vi "Find Fiducials.vi"(7 "Console Log in":refnum<class "Console Log.lvclass">, 8 "error in":errorcluster, 11 "Potting Procedure in":refnum<class "Potting Procedure.lvclass">) -> (0 "error out":errorcluster, 3 "Potting Procedure out":refnum<class "Potting Procedure.lvclass">, 5 "Console Log out":refnum<class "Console Log.lvclass">)   [LabVIEW 2011, in "Potting Procedure.lvclass"]
uses:
  Potting Procedure.lvclass
  UI Classes/Console Log/Console Log.lvclass
  Shared Components/Utils/Type Definitions/Fiducial Image.ctl
  Shared Components/Utils/Type Definitions/Physical Image.ctl
  Shared Components/Vec3d Class/Vec3d Class.lvclass
  <vilib>/vision/Image Controls.llb/IMAQ Image.ctl
  Shared Components/Utils/Type Definitions/Fiducial with Source.ctl
  Type Definitions/Find Fiducials.ctl
  Potting Procedure.lvclass/Potting Procedure.ctl
  Shared Components/Gantry Class/Gantry Class.lvclass
  Shared Components/WorkTable Class/WorkTable Class.lvclass
  Shared Components/CameraTool Class/CameraTool Class.lvclass
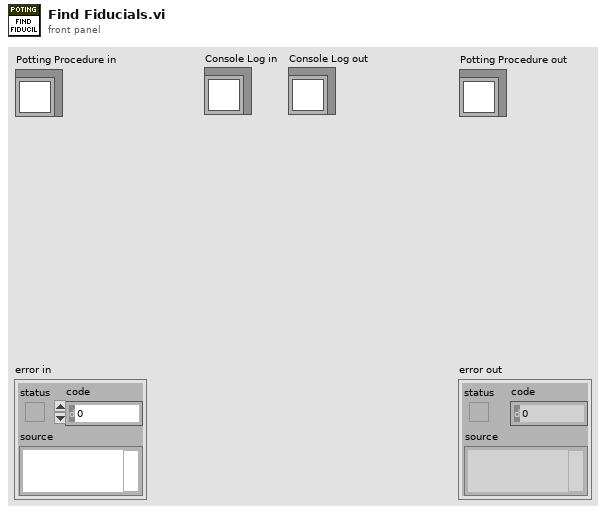
[diagram p1: front panel]
types:
  T1 = typedef "Fiducial Image.ctl" = cluster{"Fiducial Image":T2, "Selected Fiducial":T4}
  T2 = typedef "Physical Image.ctl" = cluster{"Image Position":refnum<class "Vec3d Class.lvclass">, "Image Reference":T3, "Field of View":cluster{"x(mm)":dbl, "y(mm)":dbl}}
  T3 = typedef "IMAQ Image.ctl" = refnum<image>
  T4 = typedef "Fiducial with Source.ctl" = cluster{"Fiducial Image Coordinate":refnum<class "Vec3d Class.lvclass">, "Fiducial Source":enum16{"Pattern Recognition", "User", "Error"}}
  T5 = cluster{"Fiducials-HDI":T1[], "Fiducials-BBM":T1[], "Chuck":i32, "Slot":i32}[]
  T6 = typedef "Find Fiducials.ctl" = cluster{"Has Been Run?":bool, "Module-Chuck Fiducials":cluster{"Fiducials-HDI":T1[], "Fiducials-BBM":T1[], "Chuck":i32, "Slot":i32}[]}
  T7 = enum16{"Empty", "Unglued", "Stamped", "PartOnTop", "Weighted", "Unpotted", "Potted"}
  T8 = cluster{"Fiducials-HDI":T1[], "Fiducials-BBM":T1[], "Chuck":i32, "Slot":i32}
  T9 = typedef "Worktable_Module Slot.ctl" = cluster{"Slot State":enum16{"Empty", "Unglued", "Stamped", "PartOnTop", "Weighted", "Unpotted", "Potted"}, "BBM Type":enum16{"None", "BBM", "GlassSlide"}, "HDI Type":enum16{"None", "HDI", "Polyimide"}, "Vacuum Channel":u8, "Location/Orientation BBM":T10, "Location/Orientation HDI":T10, "S/N":string}
  T10 = typedef "Position_Orientation.ctl" = cluster{"Center":refnum<class "Vec3d Class.lvclass">, "Orientation":refnum<class "Orient3d Class.lvclass">}
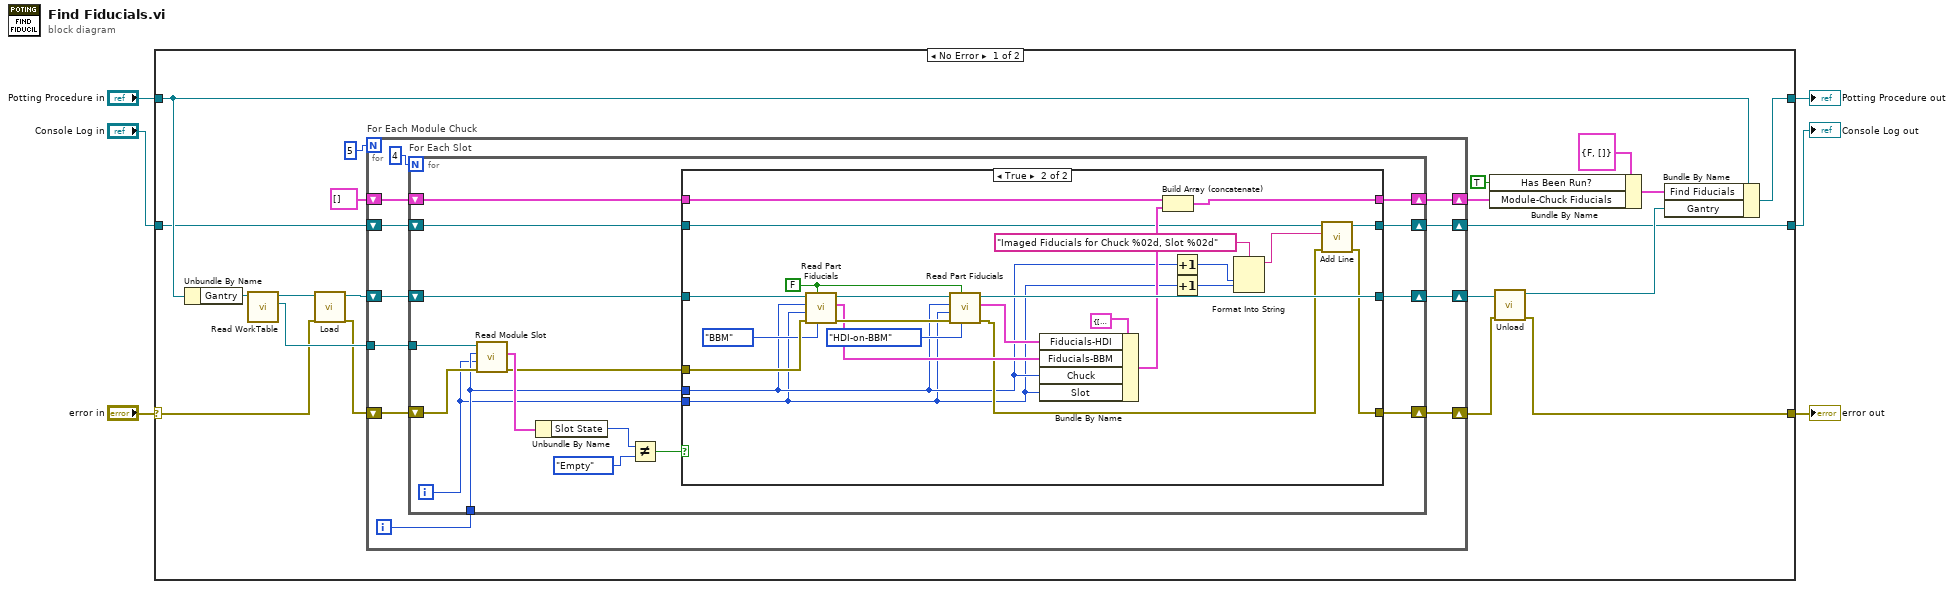
[diagram p0: block diagram]
diagram:
  n1 = case shown="No Error" "error in" {
    selector: "error in" -> [w18 w84]
    tunnel: [w14 w84] -> w5
    tunnel: [w13 w83] -> w3
    tunnel: "Potting Procedure in" -> [w16 w83]
    tunnel: "Console Log in" -> [w10 w82]
    tunnel: [w9 w82] -> w1
    frame No Error {
      n2 = Unbundle By Name(w16) -> ("Gantry"=w26:refnum<class "Gantry Class.lvclass">)
      n3 = call-dynamic "Read WorkTable.vi"("Gantry Class in"=w26) -> ("WorkTable Class.lvclass"=w24:refnum<class "WorkTable Class.lvclass">, "Gantry Class out"=w25:refnum<class "Gantry Class.lvclass">)  [unwired: 8 in, 1 out]
      n4 = call "Load.vi"("error in"=w18, "Gantry In"=w25) -> ("error out"=w22:errorcluster, "CameraTool out"=w21:refnum<class "CameraTool Class.lvclass">)  [unwired: 8 in]
      n5 = for "For Each Module Chuck" {
        N: 5 -> [_]
        tunnel: w24 -> [w37]
        shift-right: [w32] -> w17
        shift-left: w21 -> [w33]
        shift-right: [w31] -> w15
        shift-left: w22 -> [w35]
        shift-right: [w29] -> w7
        shift-left: T5 [] ("Module-Chuck Fiducials") -> [w30]
        shift-right: [w27] -> w9
        shift-left: w10 -> [w28]
        i -> [w34]
        n6 = for "For Each Slot" {
          N: 4 -> [_]
          tunnel: w37 -> [w53]
          tunnel: w34 -> [w46]
          shift-right: [w43] -> w32
          shift-left: w33 -> [w47]
          shift-right: [w42] -> w31
          shift-left: w35 -> [w52]
          shift-right: [w40] -> w29
          shift-left: w30 -> [w41]
          shift-right: [w38] -> w27
          shift-left: w28 -> [w39]
          i -> [w45]
          n7 = call-dynamic "Read Module Slot.vi"("error in"=w52, "slot"=w45, "chuck"=w46, "WorkTable in"=w53) -> ("error out"=w44:errorcluster, "Module Slot"=w51:T9)  [unwired: 5 in, 1 out]
          n8 = Unbundle By Name(w51) -> ("Slot State"=w49:T7)
          n9 = Not Equal?(x=w49, y=T7."Empty" ("BBM Slot State")) -> (x != y?=w48:bool)
          n10 = case shown="True" w48 {
            tunnel: w47 -> [w57 w81]
            tunnel: w46 -> [_ w60]
            tunnel: w45 -> [_ w59]
            tunnel: w44 -> [w56 w80]
            tunnel: [w57 w72] -> w43
            tunnel: [w56 w65] -> w42
            tunnel: w41 -> [w55 w71]
            tunnel: [w55 w69] -> w40
            tunnel: w39 -> [w54 w68]
            tunnel: [w54 w67] -> w38
            frame False {
            }
            frame True {
              w77 = FALSE ("Dispose Images?")
              n11 = call-dynamic "Read Part Fiducials.vi"("Part Type"=enum16{"HDI", "BBM", "HDI-on-BBM"}."BBM", "Dispose Images?"=w77, "error in"=w80, "Slot"=w59, "Chuck"=w60, "CameraTool in"=w81) -> ("error out"=w76:errorcluster, "Fiducials"=w73:T1[], "CameraTool out"=w78:refnum<class "CameraTool Class.lvclass">)  [unwired: 3 in]
              n12 = call-dynamic "Read Part Fiducials.vi"("Part Type"=enum16{"HDI", "BBM", "HDI-on-BBM"}."HDI-on-BBM", "Dispose Images?"=w77, "error in"=w76, "Slot"=w59, "Chuck"=w60, "CameraTool in"=w78) -> ("error out"=w66:errorcluster, "Fiducials"=w74:T1[], "CameraTool out"=w72:refnum<class "CameraTool Class.lvclass">)  [unwired: 3 in]
              n13 = Bundle By Name(cluster=T8 {"Fiducials-HDI"=[], "Fiducials-BBM"=[], "Chuck"=0, "Slot"=0} ("Module Fiducials"), "Fiducials-HDI"=w74, "Fiducials-BBM"=w73, "Chuck"=w60, "Slot"=w59) -> (w70:T8)
              n14 = Build Array (concatenate)(w71, w70) -> (w69:T5)
              n15 = Increment(x=w60) -> (x+1=w62:i32)
              n16 = Increment(x=w59) -> (x+1=w61:i32)
              n17 = Format Into String(format string="Imaged Fiducials for Chuck %02d, Slot %02d", w62, w61) -> (resulting string=w64:string)  [unwired: 2 in, 1 out]
              n18 = call "Add Line.vi"("error in (no error)"=w66, "String"=w64, "Console Log in"=w68) -> ("error out"=w65:errorcluster, "Console Log out"=w67:refnum<class "Console Log.lvclass">)  [unwired: 7 in]
            }
          }
        }
      }
      n19 = Bundle By Name(cluster=T6 {"Has Been Run?"=FALSE, "Module-Chuck Fiducials"=[]} ("Find Fiducials"), "Has Been Run?"=TRUE, "Module-Chuck Fiducials"=w7) -> (w11:T6)
      n20 = call "Unload.vi"("error in (no error)"=w15, "CameraTool in"=w17) -> ("error out"=w14:errorcluster, "Gantry out"=w12:refnum<class "Gantry Class.lvclass">)  [unwired: 8 in]
      n21 = Bundle By Name(cluster=w16, "Find Fiducials"=w11, "Gantry"=w12) -> (w13:refnum<class "Potting Procedure.lvclass">)
    }
    frame Error {
    }
  }
  "error out" <- w5
  "Potting Procedure out" <- w3
  "Console Log out" <- w1
